vi "Chroma 1905x Series Configure Dwell Time Query.vi"(7 "Mode":T2 items=["DC", "IR"], 8 "error in (no error)":errorcluster, 10 "Step":T1=1 min=1 max=99 step=1, 11 "VISA resource name":refnum<visa-resource-name>) -> (0 "error out":errorcluster, 2 "Dwell time value [s]":string, 3 "VISA resource name out":refnum<visa-resource-name>)   [LabVIEW 2025]
uses:
  Type Def/DC-IR modes--ring.ctl
  Type Def/steps--numeric.ctl
panel:
  # "Dwell Time query"
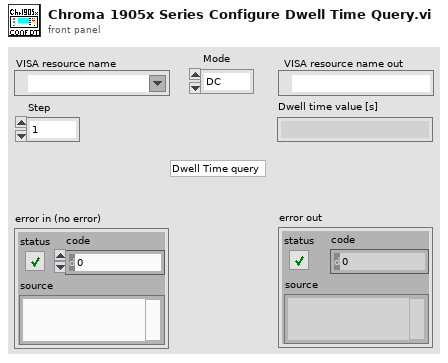
[diagram p1: front panel]
types:
  T1 = typedef "steps--numeric.ctl" = u8
  T2 = typedef "DC-IR modes--ring.ctl" = u16
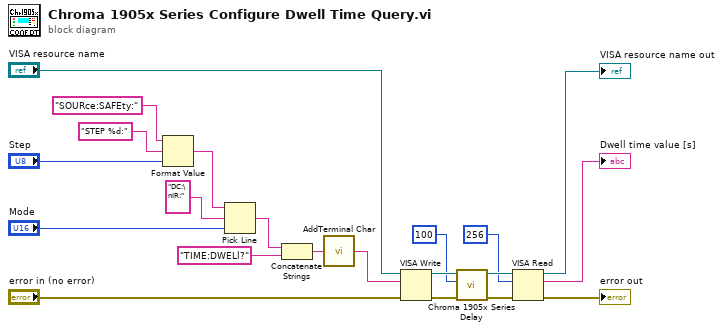
[diagram p0: block diagram]
diagram:
  n1 = Format Value(string ("")="SOURce:SAFEty:", format string="STEP %d:", value (0)="Step") -> (output string=w16:string)
  n2 = Pick Line(string ("")=w16, multi-line string="DC:\nIR:", line index="Mode") -> (output string=w14:string)
  n3 = Concatenate Strings(w14, "TIME:DWELl?" ("format string")) -> (w15:string)
  n4 = call "AddTerminal Char.vi"("Cmd string"=w15) -> ("Concatenated String"=w5:string)  [unwired: 4 in]
  n5 = VISA Write(VISA resource name="VISA resource name", write buffer=w5, error in (no error)="error in (no error)") -> (VISA resource name out=w10:refnum<visa-resource-name>, error out=w12:errorcluster)  [unwired: 1 out]
  n6 = call "Chroma 1905x Series Delay.vi"("error in (no error)"=w12, "Time Delay [ms]"=u32 100 ("Time Delay ms"), "VISA resource name"=w10) -> ("error out"=w11:errorcluster, "VISA resource name 2"=w9:refnum<visa-resource-name>)  [unwired: 7 in]
  n7 = VISA Read(VISA resource name=w9, byte count=u32 256, error in (no error)=w11) -> (VISA resource name out=→"VISA resource name out":refnum<visa-resource-name>, read buffer=→"Dwell time value [s]":string, error out=→"error out":errorcluster)  [unwired: 1 out]
